vi "Angles_nano.vi"() -> (1 "psi":dbl, 2 "phi":dbl, 3 "theta":dbl)   [LabVIEW 2017]
uses:
  Program Files/National Instruments/LabVIEW 2019/user.lib/HapticSTM/HapticSTM.lvlib
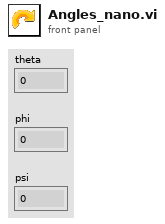
[diagram p1: front panel]
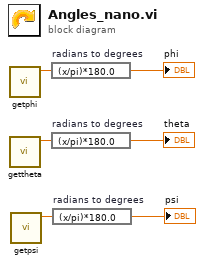
[diagram p0: block diagram]
diagram:
  n1 = call "getphi.vi"() -> ("function return"=w4:dbl)  [unwired: 11 in]
  n2 = call "gettheta.vi"() -> ("function return"=w6:dbl)  [unwired: 11 in]
  n3 = call "getpsi.vi"() -> ("function return"=w2:dbl)  [unwired: 11 in]
  n4 = expression code="(x/pi)*180.0" "radians to degrees"(w4) -> (→"phi":dbl)
  n5 = expression code="(x/pi)*180.0" "radians to degrees"(w6) -> (→"theta":dbl)
  n6 = expression code="(x/pi)*180.0" "radians to degrees"(w2) -> (→"psi":dbl)
